vi "new http responder.vi"(8 "error in":errorcluster, 11 "http responder in":refnum<class "http responder.lvclass">) -> (0 "error out":errorcluster, 3 "http responder out":refnum<class "http responder.lvclass">)   [LabVIEW 2013, in "http responder.lvclass"]
uses:
  http responder.lvclass
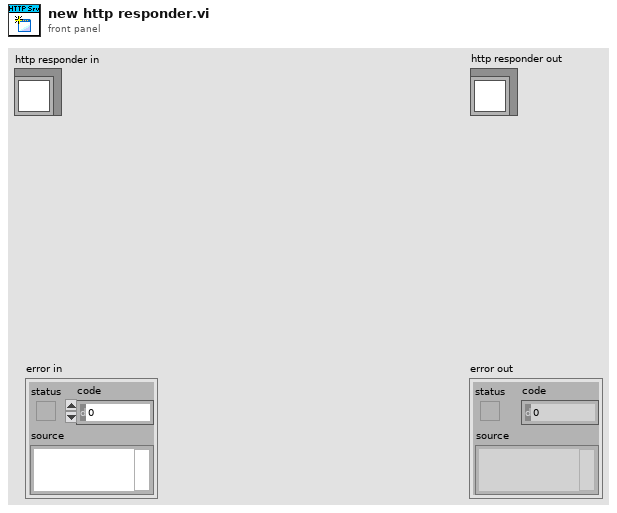
[diagram p1: front panel]
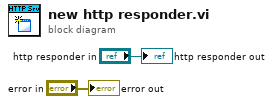
[diagram p0: block diagram]
diagram:
  "error out" <- "error in"
  "http responder out" <- "http responder in"
